vi "light curtain test.vi"() -> ()   [LabVIEW 2021, in "Test VIs.lvclass"]
uses:
  Test VIs.lvclass
  Classes/Controller/I-O/I-O.lvclass
  Classes/Controller/Controller.lvclass
panel:
  in  "stop":bool
  out "error out":errorcluster
  out "Curtain Broken?":bool
  in  "error in (no error)":errorcluster
  out "Dispenser error?":bool
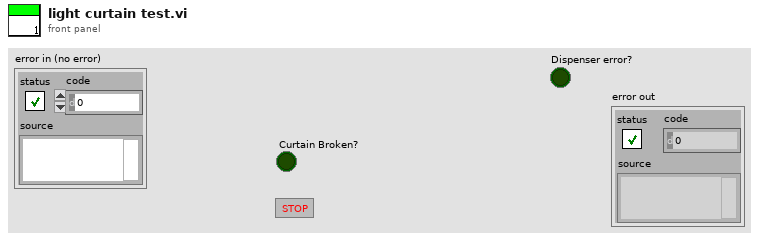
[diagram p1: front panel]
types:
  T1 = typedef "Controller.lvclass/Controllers.ctl" = cluster{"I-O.lvclass":refnum<class "I-O.lvclass">, "Gantry":refnum<k24>, "Dispenser":refnum<visa-resource-name>}
  T2 = typedef "I-O.lvclass/Pin Map.ctl" = cluster{"Region Valves":i32[], "Extra Valves":dbl[][][], "Tool Primary Valve":i32, "Tool Secondary Valve":i32, "Region Sensors":i32[], "Extra Sensors":dbl[][][], "Tool Primary Sensor":dbl, "Tool Secondary Sensor":dbl, "Compression Sensor":dbl, "5V":i32, "Dispenser Sensor":dbl, "Light Curtain":i32}
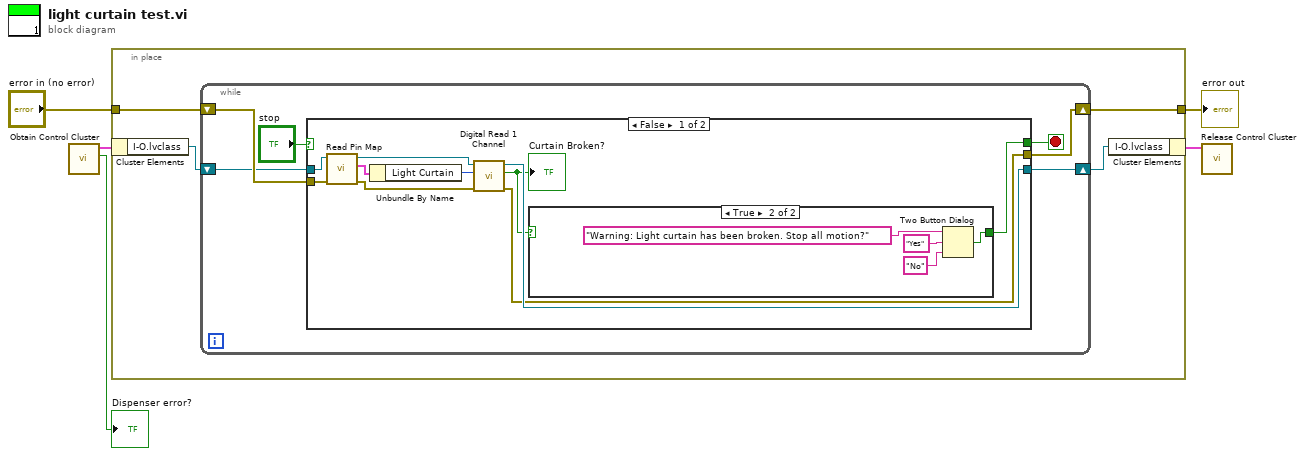
[diagram p0: block diagram]
diagram:
  n1 = call "Obtain Control Cluster.vi"() -> ("Dispenser error?"=→"Dispenser error?":bool, "Control Out"=w3:T1)  [unwired: 10 in]
  n2 = in-place {
    in-place-border: "error in (no error)" -> [w9]
    in-place-border: [w6] -> w1
    n3 = in-place-cluster #1(w3) -> ("I-O.lvclass"=w8:refnum<class "I-O.lvclass">)
    n4 = while {
      shift-right: [w13] -> w7
      shift-left: w8 -> [w14]
      shift-right: [w12] -> w6
      shift-left: w9 -> [w15]
      stop <- w11 stop-if-true
      n5 = case shown="False" "stop" {
        selector: "stop" -> [_ w33]
        tunnel: w15 -> [w21 w32]
        tunnel: w14 -> [w20 w31]
        tunnel: [w19 w31] -> w13
        tunnel: [w18 w32] -> w12
        tunnel: [w16 w33] -> w11
        frame False {
          n6 = call-dynamic "Read Pin Map.vi"("error in (no error)"=w21, "I-O in"=w20) -> ("error out"=w22:errorcluster, "Pin Map 2"=w24:T2, "I-O out"=w25:refnum<class "I-O.lvclass">)  [unwired: 7 in]
          n7 = Unbundle By Name(w24) -> ("Light Curtain"=w23:i32)
          n8 = call-dynamic "Digital Read 1 Channel.vi"("error in (no error)"=w22, "Read"=w23, "I-O in"=w25) -> ("error out"=w18:errorcluster, "Value"=w17:bool, "I-O out"=w19:refnum<class "I-O.lvclass">)  [unwired: 6 in]
          "Curtain Broken?" <- w17
          n9 = case shown="True" w17 {
            selector: w17 -> [w26 _]
            tunnel: [w26 w29] -> w16
            frame False {
            }
            frame True {
              n10 = Two Button Dialog(message="Warning: Light curtain has been broken. Stop all motion?", 1:"No" ("F button name (\"Cancel\")"), 2:"Yes" ("message")) -> (T button?=w29:bool)
            }
          }
        }
        frame True {
        }
      }
    }
    n11 = in-place-cluster #1("I-O.lvclass"=w7) -> (w2:T1)
  }
  "error out" <- w1
  n12 = call "Release Control Cluster.vi"("output cluster"=w2) -> ()  [unwired: 11 in]
